vi "Model_Torque_Calculation2022.vi"() -> ()   [LabVIEW 2019]
uses:
  <vilib>/imath/engines/lvmath2/RunTimeEngine/NodeEndStatement/NIMS_NodeEndStatement_Output.vi
  <instcachedir>/0/NIMS_NodeEndStatement_Output_53EC0D466D134D7ABD903AC30B43404B.lvgen/NIMS_NodeEndStatement_Output_53EC0D466D134D7ABD903AC30B43404B_001.vi
  <vilib>/imath/engines/lvmath2/RunTimeEngine/ErrorHandling/NIMS_Finalize Error.vi
  <vilib>/addons/database/Connection.llb/DB Tools Open Connec (String).vi
  <vilib>/addons/database/NI_Database_API.lvlib
panel:
  in  "Reset DataBase Torque":bool
  in  "Reset DataBase length":bool
  in  "Reset DataBase Mass":bool
  out "Mass Chart":dynamicdata(graph)
  out "Joint Mass & Center Mass":string[][](array[string])
  in  "stop 2":bool
  in  "stop 3":bool
  out "segment length lower extremity":dynamicdata(graph)
  out "Length Segment":string[][](array[string])
  out "Torque Joint Chart":dynamicdata(graph)
  out "Torque Ankle Chart":dbl(graph)
  out "Torque Knee Chart":dbl(graph)
  out "Torque Hip Chart":dbl(graph)
  in  "stop":bool
  out "Torque":string[][](array[string])
  out "Data Brushed Motors":string[][](array[string])
  out "Data Brushless Motors":string[][](array[string])
  in  "Select Mass of Actuator at ankle joint":dbl(slide) scale=200.0..2200.0 scale format="%#_6f"
  in  "Select Mass of Actuator at knee joint":dbl(slide) scale=200.0..2200.0 scale format="%#_6f"
  in  "Select Mass of Actuator at hip joint":dbl(slide) scale=200.0..2200.0 scale format="%#_6f"
  out "lower leg(l2)":dbl(slide) scale=8.0..60.0
  out "foot(l3)":dbl(slide) scale=2.0..20.0
  out "thigh(l1)":dbl(slide) scale=8.0..60.0
  out "Tknee":dbl(slide) scale=-100.0..200.0
  out "Tankle":dbl(slide) scale=-10.0..10.0
  out "Thip":dbl(slide) scale=-200.0..200.0
  in  "?":dbl(slide) scale=40.0..220.0
  in  "Ankle_è3":dbl(slide) scale=-45.0..45.0
  in  "Knee_è2":dbl(slide) scale=0.0..145.0
  in  "hip_è1":dbl(slide) scale=-10.0..145.0
  in  "Select Model BSP":bool
  in  "Select sex":bool
  out "KneeD_m4":dbl(slide) scale=0.0..35.0
  out "FootD_m3":dbl(slide) scale=0.0..4.0
  out "LowerLegD_m2":dbl(slide) scale=0.0..10.0
  out "ThighD_m1":dbl(slide) scale=0.0..25.0 scale format="%#.8g"
  in  "Select Total Body mass":dbl(slide) scale=20.0..170.0
  # "CALCULATION OF BASIC SIZES OF ROBOTIC EXTRACTUAL LOWER LIMB"
  # "KINEMATIC ANALYSIS"
  # "DataBase Model                                                                        I. (Import of characteristic motor from the database)"
  # "Á.Calculate the mass of each member of the lower limb                                           in relation to its total mass"
  # "A/A"
  # "PartNo"
  # "Torque(mNm)"
  # "Weight(gr)"
  # "Power(W)"
  # "Speed(rpm)"
  # "Voltage(V)"
  # "Price(€)"
  # "Select Total Body Mass(Kg)"
  # "Select Mass Brushless or Brushed Motor(gr)"
  # "Mass Segment Body to Model Dempster or Ztsiorsky BSP"
  # "Zatsiorsky BSP as modified by de Leva"
  # "Dempster BSP"
  # "Males"
  # "A/A"
  # "PartNo"
  # "Torque(mNm)"
  # "Weight(gr)"
  # "Power(W)"
  # "Speed(rpm)"
  # "Voltage(V)"
  # "Price(€)"
  # "Female"
  # "B.Calculation of moments of each segment  of the lower right extremity in relation                                                                  to the total mass (kg) its height (m) and the change of angles of each joints."
  # "DataBase Model                                                                                                                                                                                                                                                                                                                                                                                                                                                                      II.(Input to the database of calculated moments at the lower extremity joints)"
  # "Settings force balance diagram"
  # "Results force balance diagram"
  # "Torque joint(Nm)"
  # "Select Height(cm)"
  # "Select Angles(cm)"
  # "Flexion/extension"
  # "Date"
  # "Torque Hip"
  # "Torque Knee"
  # "Torque Ankle"
  # "Date"
  # "Total Mass tm"
  # "Thigh CM_m1 CM_m2"
  # "LowerLeg CM_m2"
  # "Foot CM_m3"
  # "Knee Mass_m4"
  # "Date"
  # "Heigth"
  # "Thigh l1"
  # "Lower Leg l2"
  # "Foot l3"
  # "Length(cm)"
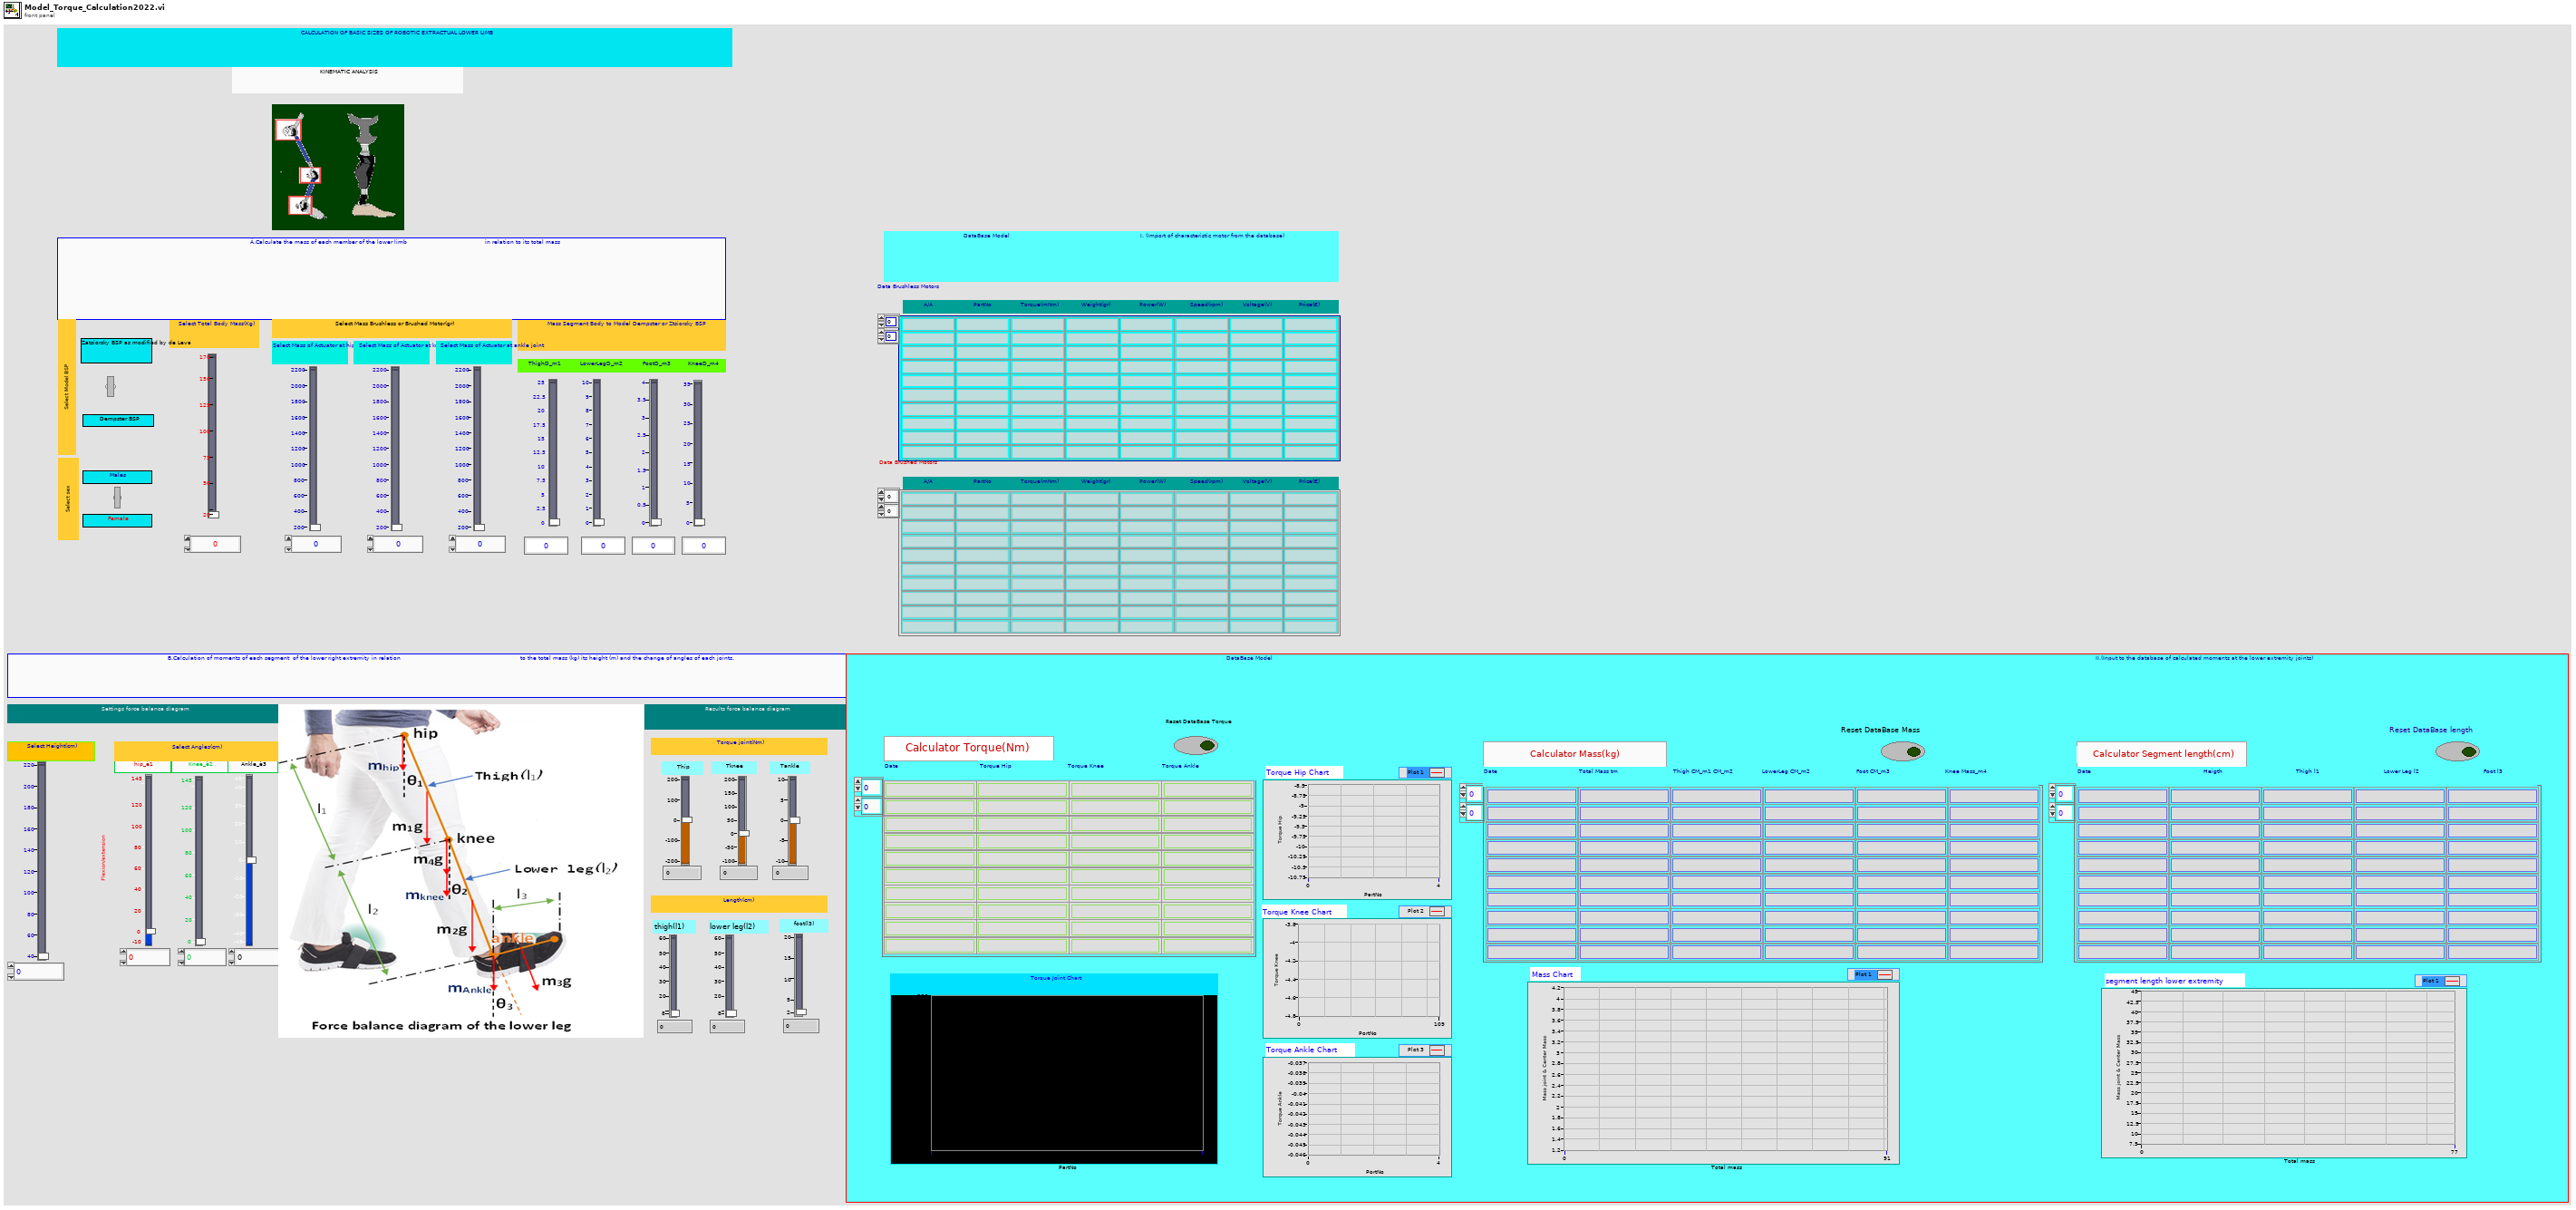
[diagram p1: front panel]
types:
  T1 = typedef "NI_Database_API.lvlib/Conn ObjectReference.ctl" = refnum<k1>
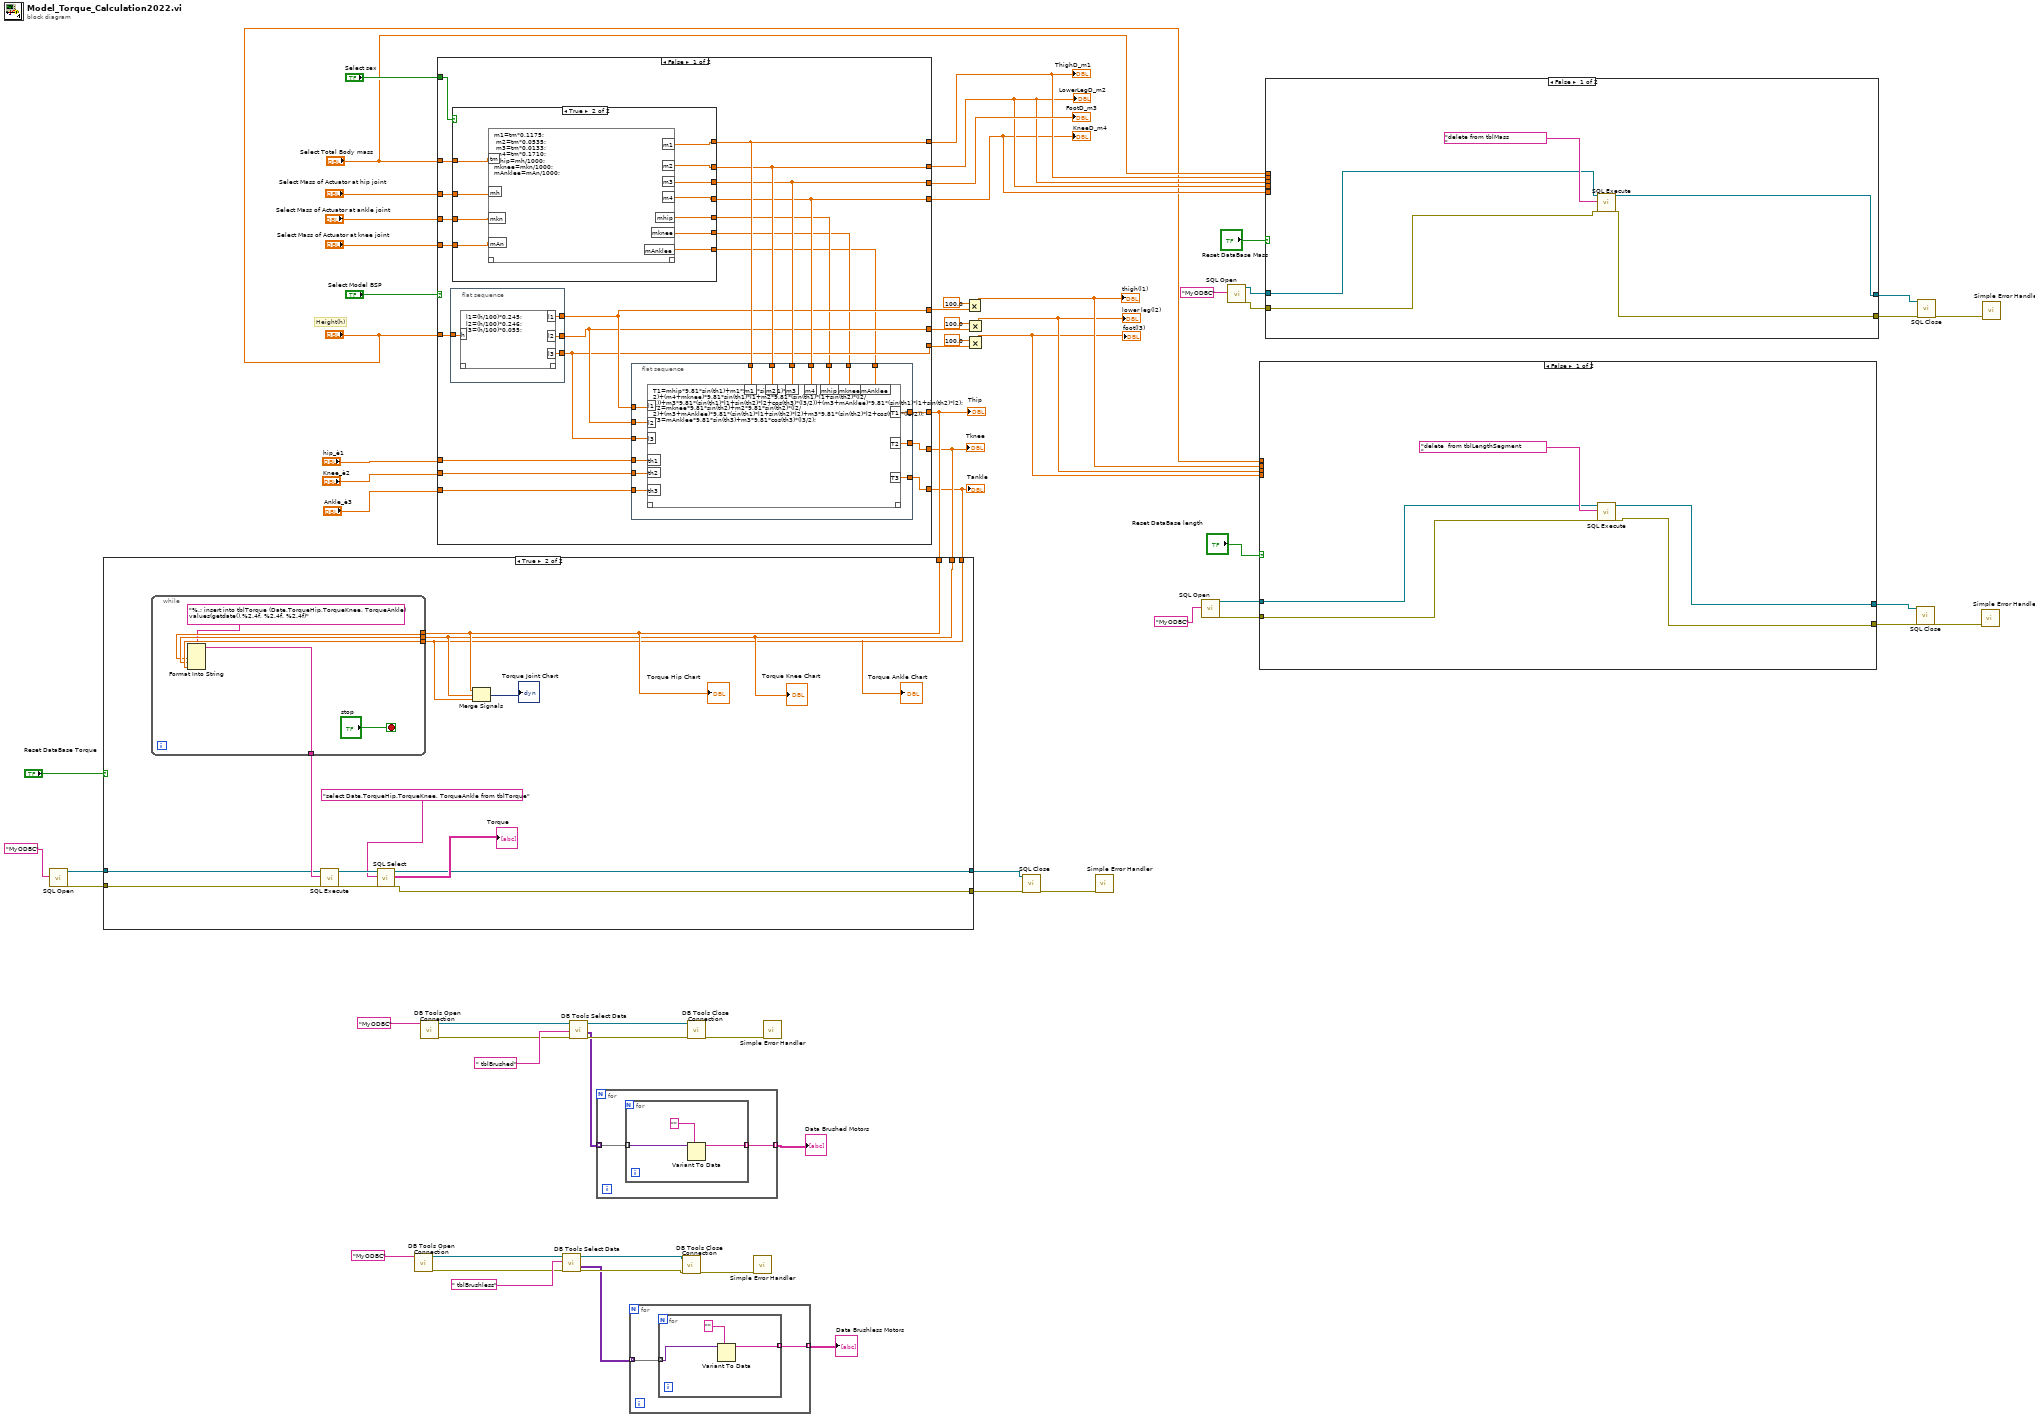
[diagram p0: block diagram]
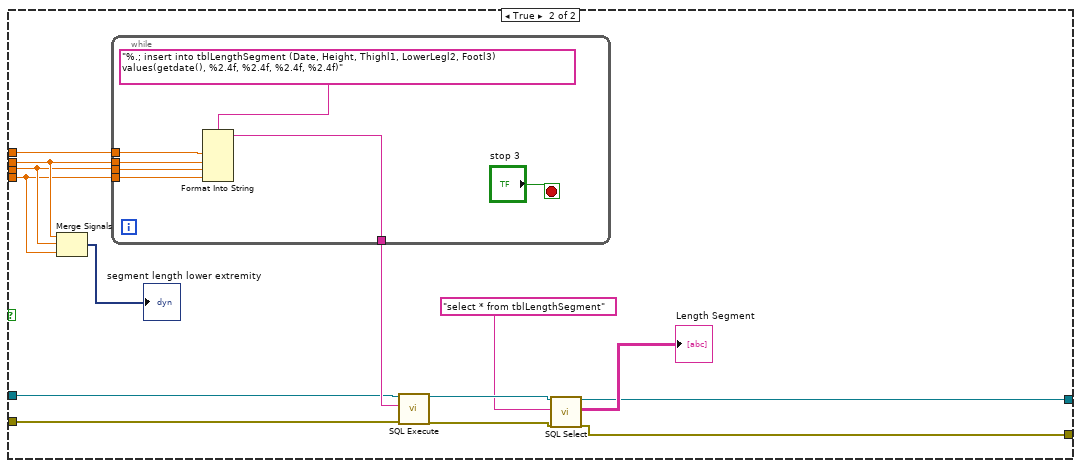
[diagram p2: hidden frame]
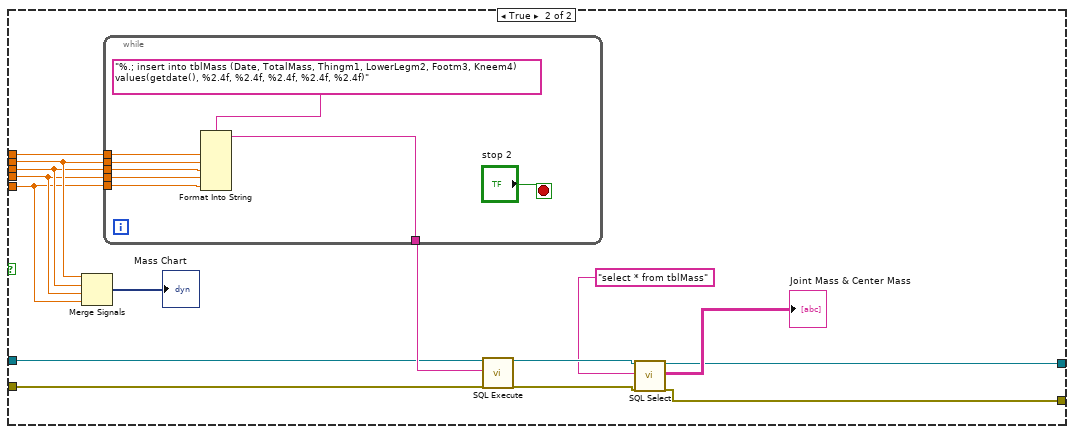
[diagram p3: hidden frame]
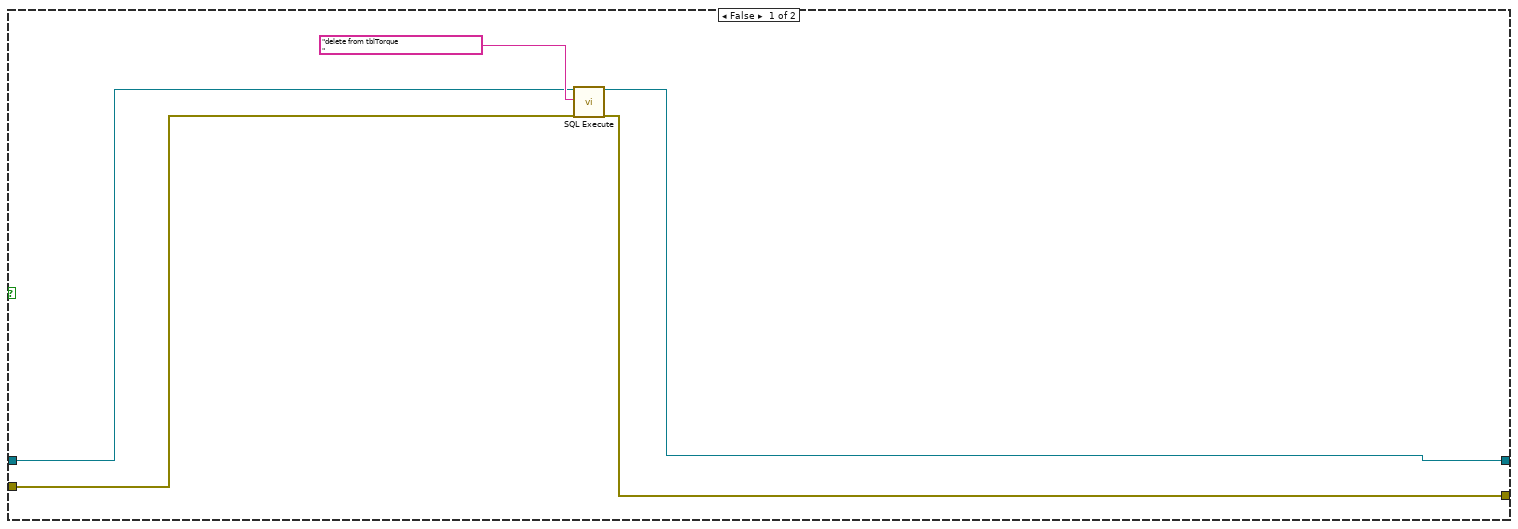
[diagram p4: hidden frame]
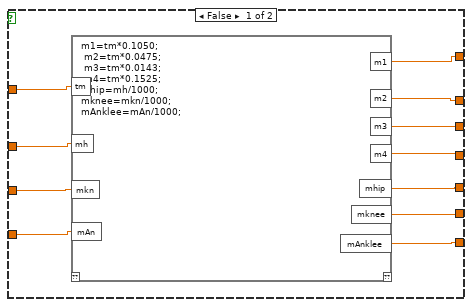
[diagram p5: hidden frame]
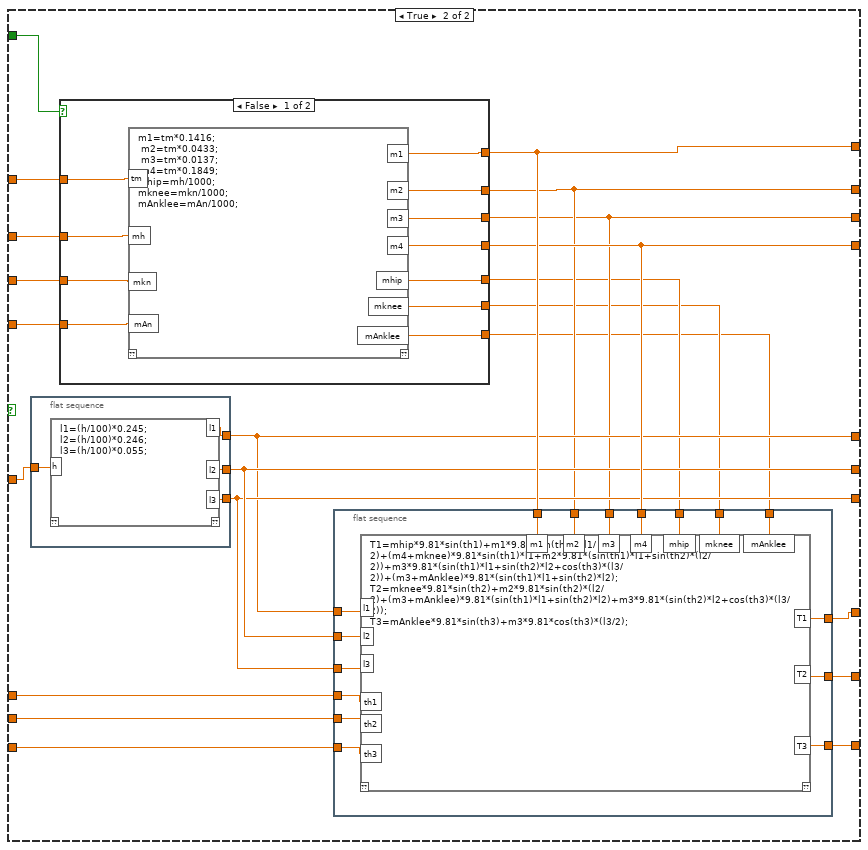
[diagram p6: hidden frame]
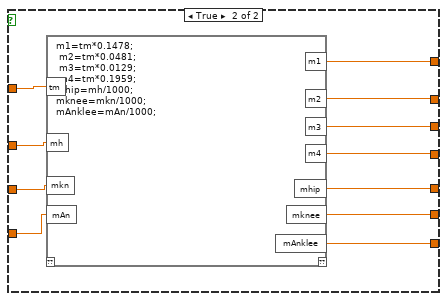
[diagram p7: hidden frame]
diagram:
  # "Height(h)"
  n1 = call <vilib>:"SQL Open.vi"("ConnectionString In"="MyODBC") -> ("Connection Out"=w19:refnum<k7>, "Error out"=w18:errorcluster)  [unwired: 17 in]
  n2 = call-poly <vilib>:"DB Tools Open Connection.vi"("connection information"="MyODBC") -> ("error out"=w38:errorcluster, "connection reference"=w39:T1)  [unwired: 7 in]
  n3 = call-poly <vilib>:"DB Tools Open Connection.vi"("connection information"="MyODBC") -> ("error out"=w45:errorcluster, "connection reference"=w46:T1)  [unwired: 7 in]
  n4 = case shown="False" "Select Model BSP" {
    tunnel: "Select sex" -> [w87 w522]
    tunnel: "Select Total Body mass" -> [w86 w521]
    tunnel: [w84 w516] -> w29
    tunnel: [w83 w508] -> w28
    tunnel: [w82 w507] -> w30
    tunnel: [w81 w515] -> w27
    tunnel: "?" -> [w85 w520]
    tunnel: "hip_è1" -> [w80 w519]
    tunnel: "Knee_è2" -> [w79 w518]
    tunnel: "Ankle_è3" -> [w78 w517]
    tunnel: [w77 w514] -> w33
    tunnel: [w76 w513] -> w32
    tunnel: [w75 w512] -> w31
    tunnel: [w73 w511] -> w56
    tunnel: [w72 w510] -> w55
    tunnel: [w74 w509] -> w60
    tunnel: "Select Mass of Actuator at hip joint" -> [w71 w506]
    tunnel: "Select Mass of Actuator at ankle joint" -> [w70 w505]
    tunnel: "Select Mass of Actuator at knee joint" -> [w69 w504]
    frame False {
      n5 = flat-sequence {
        tunnel: w85 -> [w283]
        tunnel: [w282] -> w74
        tunnel: [w281] -> w73
        tunnel: [w280] -> w72
        frame #0 {
          n6 = mathscript code="l1=(h/100)*0.245;\nl2=(h/100)*0.246;\nl3=(h/100)*0.055;"("h"=w283) -> ("l1"=w282:dbl, "l2"=w281:dbl, "l3"=w280:dbl)  [unwired: 1 in, 1 out]
        }
      }
      n7 = case shown="True" w87 {
        tunnel: [w328 w420] -> w81
        tunnel: [w329 w421] -> w82
        tunnel: [w330 w422] -> w83
        tunnel: w86 -> [w335 w419]
        tunnel: [w331 w423] -> w84
        tunnel: w71 -> [w334 w418]
        tunnel: w70 -> [w333 w417]
        tunnel: w69 -> [w332 w416]
        tunnel: [w327 w415] -> w68
        tunnel: [w326 w414] -> w67
        tunnel: [w325 w413] -> w66
        frame False {
          n8 = mathscript code="m1=tm*0.1050;\n m2=tm*0.0475;\n m3=tm*0.0143;\n m4=tm*0.1525;\nmhip=mh/1000;\nmknee=mkn/1000;\nmAnklee=mAn/1000;"("tm"=w335, "mh"=w334, "mkn"=w333, "mAn"=w332) -> ("m1"=w331:dbl, "m2"=w330:dbl, "m3"=w329:dbl, "m4"=w328:dbl, "mhip"=w327:dbl, "mknee"=w326:dbl, "mAnklee"=w325:dbl)  [unwired: 1 in, 1 out]
        }
        frame True {
          n9 = mathscript code="m1=tm*0.1175;\n m2=tm*0.0535;\n m3=tm*0.0133;\n m4=tm*0.1710;\nmhip=mh/1000;\nmknee=mkn/1000;\nmAnklee=mAn/1000;"("tm"=w419, "mh"=w418, "mkn"=w417, "mAn"=w416) -> ("m1"=w423:dbl, "m2"=w422:dbl, "m3"=w421:dbl, "m4"=w420:dbl, "mhip"=w415:dbl, "mknee"=w414:dbl, "mAnklee"=w413:dbl)  [unwired: 1 in, 1 out]
        }
      }
      n10 = flat-sequence {
        tunnel: w84 -> [w103]
        tunnel: w83 -> [w102]
        tunnel: w82 -> [w101]
        tunnel: w81 -> [w100]
        tunnel: w80 -> [w99]
        tunnel: w79 -> [w98]
        tunnel: w78 -> [w97]
        tunnel: [w96] -> w77
        tunnel: [w95] -> w76
        tunnel: [w94] -> w75
        tunnel: w74 -> [w93]
        tunnel: w73 -> [w92]
        tunnel: w72 -> [w91]
        tunnel: w68 -> [w90]
        tunnel: w67 -> [w89]
        tunnel: w66 -> [w88]
        frame #0 {
          n11 = mathscript code="T1=mhip*9.81*sin(th1)+m1*9.81*sin(th1)*(l1/2)+(m4+mknee)*9.81*sin(th1)*l1+m2*9.81*(sin(th1)*l1+sin(th2)*(l2/2))+m3*9.81*(sin(th1)*l1+sin(th2)*l2+cos(th3)*(l3/2))+(m3+mAnklee)*9.81*(sin(th1)*l1+sin(th2)*l2);\nT2=mknee*9.81*sin(th2)+m2*9.81*sin(th2)*(l2/2)+(m3+mAnklee)*9.81*(sin(th1)*l1+sin(th2)*l2)+m3*9.81*(sin(th2)*l2+cos(th3)*(l3/2));\nT3=mAnklee*9.81*sin(th3)+m3*9.81*cos(th3)*(l3/2);"("m1"=w103, "m2"=w102, "m3"=w101, "m4"=w100, "l1"=w93, "l2"=w92, "l3"=w91, "th1"=w99, "th2"=w98, "th3"=w97, "mhip"=w90, "mknee"=w89, "mAnklee"=w88) -> ("T1"=w96:dbl, "T2"=w95:dbl, "T3"=w94:dbl)  [unwired: 1 in, 1 out]
        }
      }
    }
    frame True {
      n12 = flat-sequence {
        tunnel: w520 -> [w718]
        tunnel: [w717] -> w511
        tunnel: [w716] -> w510
        tunnel: [w715] -> w509
        frame #0 {
          n13 = mathscript code="l1=(h/100)*0.245;\nl2=(h/100)*0.246;\nl3=(h/100)*0.055;"("h"=w718) -> ("l1"=w715:dbl, "l2"=w717:dbl, "l3"=w716:dbl)  [unwired: 1 in, 1 out]
        }
      }
      n14 = case shown="False" w522 {
        tunnel: [w760 w855] -> w515
        tunnel: [w761 w856] -> w507
        tunnel: [w765 w857] -> w508
        tunnel: w521 -> [w770 w858]
        tunnel: [w766 w854] -> w516
        tunnel: w506 -> [w769 w853]
        tunnel: w505 -> [w768 w852]
        tunnel: w504 -> [w767 w851]
        tunnel: [w764 w850] -> w503
        tunnel: [w763 w849] -> w502
        tunnel: [w762 w848] -> w501
        frame False {
          n15 = mathscript code="m1=tm*0.1416;\n m2=tm*0.0433;\n m3=tm*0.0137;\n m4=tm*0.1849;\nmhip=mh/1000;\nmknee=mkn/1000;\nmAnklee=mAn/1000;"("tm"=w770, "mh"=w769, "mkn"=w768, "mAn"=w767) -> ("m1"=w766:dbl, "m2"=w765:dbl, "m3"=w761:dbl, "m4"=w760:dbl, "mhip"=w764:dbl, "mknee"=w763:dbl, "mAnklee"=w762:dbl)  [unwired: 1 in, 1 out]
        }
        frame True {
          n16 = mathscript code="m1=tm*0.1478;\n m2=tm*0.0481;\n m3=tm*0.0129;\n m4=tm*0.1959;\nmhip=mh/1000;\nmknee=mkn/1000;\nmAnklee=mAn/1000;"("tm"=w858, "mh"=w853, "mkn"=w852, "mAn"=w851) -> ("m1"=w854:dbl, "m2"=w857:dbl, "m3"=w856:dbl, "m4"=w855:dbl, "mhip"=w850:dbl, "mknee"=w849:dbl, "mAnklee"=w848:dbl)  [unwired: 1 in, 1 out]
        }
      }
      n17 = flat-sequence {
        tunnel: w519 -> [w538]
        tunnel: w518 -> [w537]
        tunnel: w517 -> [w536]
        tunnel: w516 -> [w535]
        tunnel: w515 -> [w534]
        tunnel: [w533] -> w514
        tunnel: [w532] -> w513
        tunnel: [w531] -> w512
        tunnel: w511 -> [w530]
        tunnel: w510 -> [w529]
        tunnel: w509 -> [w528]
        tunnel: w508 -> [w527]
        tunnel: w507 -> [w526]
        tunnel: w503 -> [w525]
        tunnel: w502 -> [w524]
        tunnel: w501 -> [w523]
        frame #0 {
          n18 = mathscript code="T1=mhip*9.81*sin(th1)+m1*9.81*sin(th1)*(l1/2)+(m4+mknee)*9.81*sin(th1)*l1+m2*9.81*(sin(th1)*l1+sin(th2)*(l2/2))+m3*9.81*(sin(th1)*l1+sin(th2)*l2+cos(th3)*(l3/2))+(m3+mAnklee)*9.81*(sin(th1)*l1+sin(th2)*l2);\nT2=mknee*9.81*sin(th2)+m2*9.81*sin(th2)*(l2/2)+(m3+mAnklee)*9.81*(sin(th1)*l1+sin(th2)*l2)+m3*9.81*(sin(th2)*l2+cos(th3)*(l3/2));\nT3=mAnklee*9.81*sin(th3)+m3*9.81*cos(th3)*(l3/2);"("m1"=w535, "m2"=w527, "m3"=w526, "m4"=w534, "l1"=w528, "l2"=w530, "l3"=w529, "th1"=w538, "th2"=w537, "th3"=w536, "mhip"=w525, "mknee"=w524, "mAnklee"=w523) -> ("T1"=w533:dbl, "T2"=w532:dbl, "T3"=w531:dbl)  [unwired: 1 in, 1 out]
        }
      }
    }
  }
  "ThighD_m1" <- w29
  "LowerLegD_m2" <- w28
  "FootD_m3" <- w30
  "KneeD_m4" <- w27
  "Thip" <- w33
  "Tknee" <- w32
  "Tankle" <- w31
  n19 = case shown="True" "Reset DataBase Torque" {
    tunnel: w33 -> [_ w948]
    tunnel: w32 -> [_ w947]
    tunnel: w31 -> [_ w946]
    tunnel: w19 -> [w937 w944]
    tunnel: w18 -> [w936 w943]
    tunnel: [w938 w942] -> w16
    tunnel: [w939 w941] -> w15
    frame False {
      n20 = call <vilib>:"SQL Execute.vi"("Connection In"=w937, "SQL Query"="delete from tblTorque                                                                                                                       " ("string"), "Error in (no error)"=w936) -> ("Connection Out"=w938:refnum<k7>, "Error out"=w939:errorcluster)  [unwired: 15 in]
    }
    frame True {
      n21 = while {
        tunnel: w948 -> [w956]
        tunnel: w947 -> [w957]
        tunnel: w946 -> [w958]
        tunnel: [w954] -> w949
        stop <- "stop" stop-if-true
        n22 = Format Into String(format string="%.; insert into tblTorque (Date,TorqueHip,TorqueKnee, TorqueAnkle) values(getdate(),%2.4f, %2.4f, %2.4f)" ("string"), w956, w957, w958) -> (resulting string=w954:string)  [unwired: 2 in, 1 out]
      }
      n23 = call <vilib>:"SQL Execute.vi"("Connection In"=w944, "SQL Query"=w949, "Error in (no error)"=w943) -> ("Connection Out"=w951:refnum<k7>, "Error out"=w952:errorcluster)  [unwired: 15 in]
      n24 = call <vilib>:"SQL Select.vi"("Connection In"=w951, "SQL Query"="select Date,TorqueHip,TorqueKnee, TorqueAnkle from tblTorque", "Error in (no error)"=w952) -> ("Connection Out"=w942:refnum<k7>, "Data"=→"Torque":string[][], "Error out"=w941:errorcluster)  [unwired: 14 in]
      n25 = Merge Signals(w948, w947, w946) -> (→"Torque Joint Chart":dynamicdata)
      "Torque Hip Chart" <- w948
      "Torque Knee Chart" <- w947
      "Torque Ankle Chart" <- w946
    }
  }
  n26 = call <vilib>:"DB Tools Select Data.vi"("error in (no error)"=w38, "table"=" tblBrushless", "connection reference"=w39) -> ("error out"=w42:errorcluster, "data"=w37:variant[][], "connection reference out"=w41:T1)  [unwired: 3 in]
  n27 = call <vilib>:"DB Tools Select Data.vi"("error in (no error)"=w45, "table"=" tblBrushed", "connection reference"=w46) -> ("error out"=w44:errorcluster, "data"=w34:variant[][], "connection reference out"=w49:T1)  [unwired: 3 in]
  n28 = for {
    tunnel: w34 -> [w961] mode=indexing
    tunnel: [w960] -> w35 mode=indexing
    n29 = for {
      tunnel: w961 -> [w964] mode=indexing
      tunnel: [w962] -> w960 mode=indexing
      n30 = Variant To Data(type="", Variant=w964) -> (data=w962:string)  [unwired: 1 in, 1 out]
    }
  }
  "Data Brushed Motors" <- w35
  n31 = for {
    tunnel: w37 -> [w966] mode=indexing
    tunnel: [w965] -> w36 mode=indexing
    n32 = for {
      tunnel: w966 -> [w969] mode=indexing
      tunnel: [w967] -> w965 mode=indexing
      n33 = Variant To Data(type="", Variant=w969) -> (data=w967:string)  [unwired: 1 in, 1 out]
    }
  }
  "Data Brushless Motors" <- w36
  n34 = call <vilib>:"DB Tools Close Connection.vi"("error in (no error)"=w42, "connection reference"=w41) -> ("error out"=w43:errorcluster)  [unwired: 5 in]
  n35 = call <vilib>:"DB Tools Close Connection.vi"("error in (no error)"=w44, "connection reference"=w49) -> ("error out"=w50:errorcluster)  [unwired: 5 in]
  n36 = call <vilib>:"Simple Error Handler.vi"("error in (no error)"=w43) -> ()  [unwired: 4 in, 5 out]
  n37 = call <vilib>:"Simple Error Handler.vi"("error in (no error)"=w50) -> ()  [unwired: 4 in, 5 out]
  n38 = Multiply(x=100.0, y=w60) -> (x*y=w25:dbl)
  "thigh(l1)" <- w25
  n39 = Multiply(x=100.0, y=w56) -> (x*y=w24:dbl)
  "lower leg(l2)" <- w24
  n40 = Multiply(x=100.0, y=w55) -> (x*y=w23:dbl)
  "foot(l3)" <- w23
  n41 = call <vilib>:"SQL Close.vi"("Connection In"=w16, "Error in (no error)"=w15) -> ("Error out"=w17:errorcluster)  [unwired: 17 in]
  n42 = call <vilib>:"Simple Error Handler.vi"("error in (no error)"=w17) -> ()  [unwired: 4 in, 5 out]
  n43 = call <vilib>:"SQL Open.vi"("ConnectionString In"="MyODBC") -> ("Connection Out"=w8:refnum<k7>, "Error out"=w7:errorcluster)  [unwired: 17 in]
  n44 = call <vilib>:"SQL Open.vi"("ConnectionString In"="MyODBC") -> ("Connection Out"=w5:refnum<k7>, "Error out"=w4:errorcluster)  [unwired: 17 in]
  n45 = case shown="False" "Reset DataBase length" {
    tunnel: w25 -> [_ w982]
    tunnel: w24 -> [_ w981]
    tunnel: w23 -> [_ w980]
    tunnel: "?" -> [_ w979]
    tunnel: [w972 w978] -> w11
    tunnel: [w973 w977] -> w10
    tunnel: w8 -> [w971 w976]
    tunnel: w7 -> [w970 w975]
    frame False {
      n46 = call <vilib>:"SQL Execute.vi"("Connection In"=w971, "SQL Query"="delete  from tblLengthSegment                                                                                                                        " ("string"), "Error in (no error)"=w970) -> ("Connection Out"=w972:refnum<k7>, "Error out"=w973:errorcluster)  [unwired: 15 in]
    }
    frame True {
      n47 = Merge Signals(w982, w981, w980) -> (→"segment length lower extremity":dynamicdata)
      n48 = while {
        tunnel: w982 -> [w991]
        tunnel: w981 -> [w990]
        tunnel: w980 -> [w989]
        tunnel: [w993] -> w983
        tunnel: w979 -> [w992]
        stop <- "stop 3" stop-if-true
        n49 = Format Into String(format string="%.; insert into tblLengthSegment (Date, Height, Thighl1, LowerLegl2, Footl3) values(getdate(), %2.4f, %2.4f, %2.4f, %2.4f)" ("string"), w992, w991, w990, w989) -> (resulting string=w993:string)  [unwired: 2 in, 1 out]
      }
      n50 = call <vilib>:"SQL Execute.vi"("Connection In"=w976, "SQL Query"=w983, "Error in (no error)"=w975) -> ("Connection Out"=w988:refnum<k7>, "Error out"=w987:errorcluster)  [unwired: 15 in]
      n51 = call <vilib>:"SQL Select.vi"("Connection In"=w988, "SQL Query"="select * from tblLengthSegment", "Error in (no error)"=w987) -> ("Connection Out"=w978:refnum<k7>, "Data"=→"Length Segment":string[][], "Error out"=w977:errorcluster)  [unwired: 14 in]
    }
  }
  n52 = case shown="False" "Reset DataBase Mass" {
    tunnel: w29 -> [_ w1009]
    tunnel: w28 -> [_ w1008]
    tunnel: w28 -> [_ w1007]
    tunnel: w27 -> [_ w1006]
    tunnel: "Select Total Body mass" -> [_ w1005]
    tunnel: w5 -> [w999 w1004]
    tunnel: w4 -> [w998 w1003]
    tunnel: [w997 w1002] -> w2
    tunnel: [w996 w1001] -> w1
    frame False {
      n53 = call <vilib>:"SQL Execute.vi"("Connection In"=w999, "SQL Query"="delete from tblMass                                                                                                                        " ("string"), "Error in (no error)"=w998) -> ("Connection Out"=w997:refnum<k7>, "Error out"=w996:errorcluster)  [unwired: 15 in]
    }
    frame True {
      n54 = Merge Signals(w1009, w1008, w1007, w1006) -> (→"Mass Chart":dynamicdata)
      n55 = while {
        tunnel: w1009 -> [w1019]
        tunnel: w1008 -> [w1018]
        tunnel: w1007 -> [w1017]
        tunnel: w1006 -> [w1016]
        tunnel: [w1021] -> w1011
        tunnel: w1005 -> [w1020]
        stop <- "stop 2" stop-if-true
        n56 = Format Into String(format string="%.; insert into tblMass (Date, TotalMass, Thingm1, LowerLegm2, Footm3, Kneem4) values(getdate(), %2.4f, %2.4f, %2.4f, %2.4f, %2.4f)" ("string"), w1020, w1019, w1018, w1017, w1016) -> (resulting string=w1021:string)  [unwired: 2 in, 1 out]
      }
      n57 = call <vilib>:"SQL Execute.vi"("Connection In"=w1004, "SQL Query"=w1011, "Error in (no error)"=w1003) -> ("Connection Out"=w1015:refnum<k7>, "Error out"=w1014:errorcluster)  [unwired: 15 in]
      n58 = call <vilib>:"SQL Select.vi"("Connection In"=w1015, "SQL Query"="select * from tblMass", "Error in (no error)"=w1014) -> ("Connection Out"=w1002:refnum<k7>, "Data"=→"Joint Mass & Center Mass":string[][], "Error out"=w1001:errorcluster)  [unwired: 14 in]
    }
  }
  n59 = call <vilib>:"SQL Close.vi"("Connection In"=w11, "Error in (no error)"=w10) -> ("Error out"=w12:errorcluster)  [unwired: 17 in]
  n60 = call <vilib>:"SQL Close.vi"("Connection In"=w2, "Error in (no error)"=w1) -> ("Error out"=w3:errorcluster)  [unwired: 17 in]
  n61 = call <vilib>:"Simple Error Handler.vi"("error in (no error)"=w12) -> ()  [unwired: 4 in, 5 out]
  n62 = call <vilib>:"Simple Error Handler.vi"("error in (no error)"=w3) -> ()  [unwired: 4 in, 5 out]
